vi "Initialize RT Main.vi"(8 "error in (no error)":errorcluster, 11 "OnCompile Settings":T1 {"XNET Settings"."Ghost"."FD ISO Mode" items=["ISO", "Non ISO", "ISO Legacy"]; "XNET Settings"."Ghost"."CAN I/O Mode" items=["CAN 2.0", "CAN FD", "CAN FD+BRS"]; "XNET Settings"."Ghost"."Termination" items=["Off", "On"]; "XNET Settings"."Primary"."FD ISO Mode" items=["ISO", "Non ISO", "ISO Legacy"]; "XNET Settings"."Primary"."CAN I/O Mode" items=["CAN 2.0", "CAN FD", "CAN FD+BRS"]; "XNET Settings"."Primary"."Termination" items=["Off", "On"]}) -> (0 "error out":errorcluster, 2 "FPGA Session":u32, 3 "Settings":T8[](array[typedef]) {"Port Info"."FD ISO Mode" items=["ISO", "Non ISO", "ISO Legacy"]; "Port Info"."CAN I/O Mode" items=["CAN 2.0", "CAN FD", "CAN FD+BRS"]; "Port Info"."Termination" items=["Off", "On"]})   [LabVIEW 2019, in "Ghost Bus Addon Engine.lvlib"]
uses:
  Ghost Bus Addon Engine.lvlib
  Types/RT Bus Settings.ctl
  Types/RT XNET Refs.ctl
  Addon Shared/Types/XNET Port Settings.ctl
  Types/RT Filter DVR Refs.ctl
  Addon Shared/Types/Exported.OnCompile.ctl
  Addon Shared/Types/XNET Settings.ctl
  Addon Shared/Types/Exported.Bus.Settings.ctl
  Addon Shared/Types/Exported.Frames.Settings.ctl
  Addon Shared/Types/Frame Settings.ctl
  Addon Shared/Types/986x.ctl
  Bitfile.Download.vi
  <vilib>/Utility/libraryn.llb/Check if File or Folder Exists.vi
  <vilib>/Utility/error.llb/Error Cluster From Error Code.vi
  <vilib>/rvi/Utilities/XML/nirviXML_GetValue.vi
  <vilib>/rvi/Utilities/XML/nirviXML_GetValue_String.vi
  <vilib>/xnet/xnet.llb/XNET Create Session.vi
  <vilib>/xnet/xnet.llb/XNET Create Session (Frame Output Stream).vi
  <vilib>/xnet/xnet.llb/XNET Create Session (Frame Input Stream).vi
  <vilib>/xnet/xnet.llb/XNET Create Session (Conversion).vi
  Addon Shared/Ghost Bus Addon Shared.lvlib
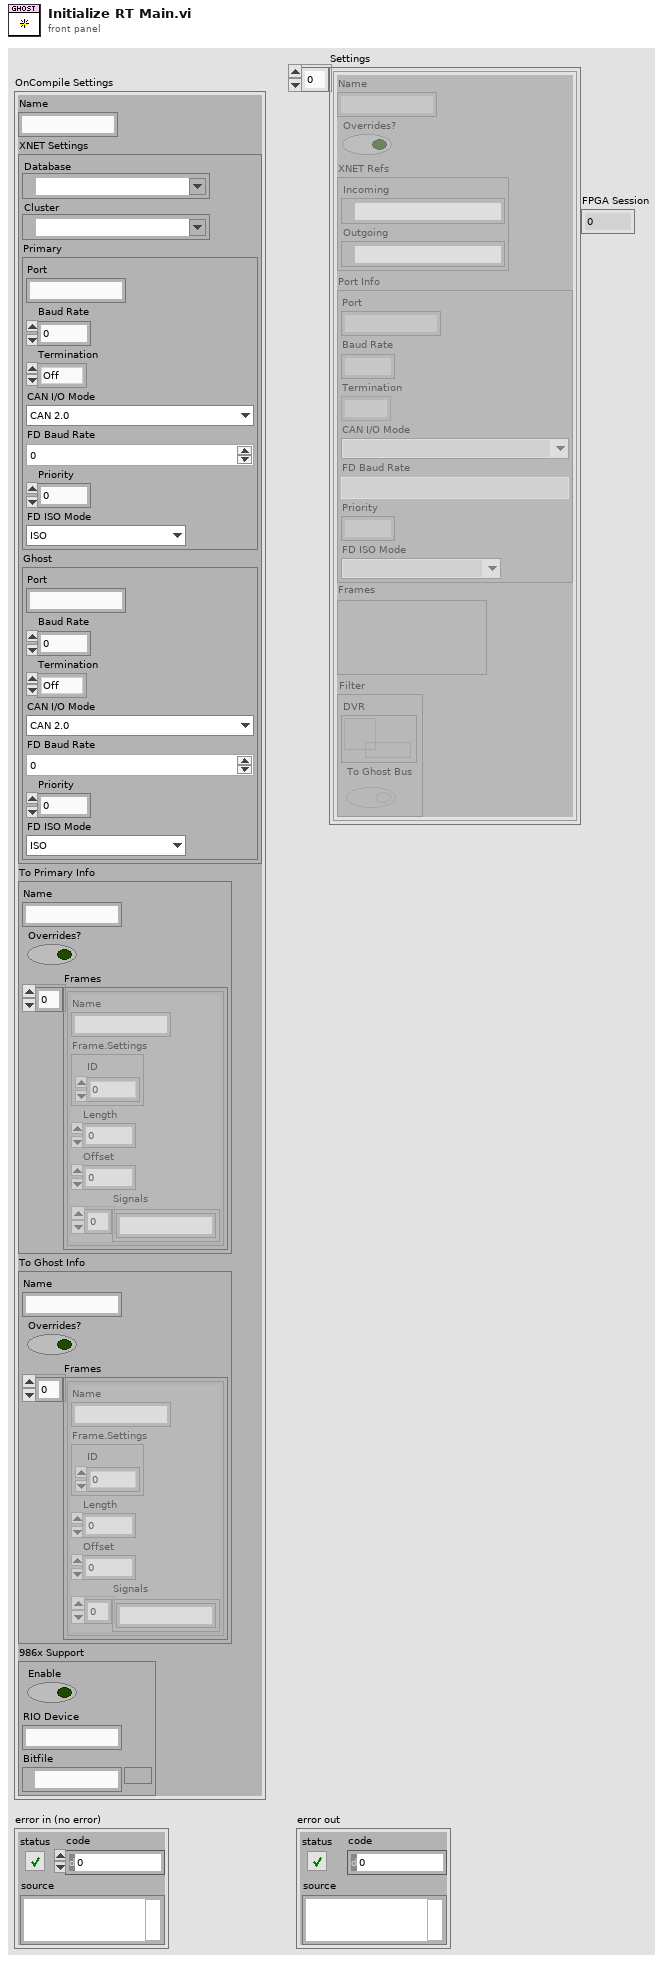
[diagram p1: front panel]
types:
  T1 = typedef "Ghost Bus Addon Shared.lvlib/Exported.OnCompile.ctl" = cluster{"Name":string, "XNET Settings":T2, "To Primary Info":T4, "To Ghost Info":T4, "986x Support":T7}
  T2 = typedef "Ghost Bus Addon Shared.lvlib/XNET Settings.ctl" = cluster{"Database":refnum<k21>, "Cluster":refnum<k21>, "Primary":T3, "Ghost":T3}
  T3 = typedef "Ghost Bus Addon Shared.lvlib/XNET Port Settings.ctl" = cluster{"Port":string, "Baud Rate":u64, "Termination":u32, "CAN I/O Mode":u32, "FD Baud Rate":u64, "Priority":i32, "FD ISO Mode":u32}
  T4 = typedef "Ghost Bus Addon Shared.lvlib/Exported.Bus.Settings.ctl" = cluster{"Name":string, "Overrides?":bool, "Frames":T5[]}
  T5 = typedef "Ghost Bus Addon Shared.lvlib/Exported.Frames.Settings.ctl" = cluster{"Name":string, "Frame.Settings":T6, "Length":i32, "Offset":i32, "Signals":string[]}
  T6 = typedef "Ghost Bus Addon Shared.lvlib/Frame Settings.ctl" = cluster{"ID":u32}
  T7 = typedef "Ghost Bus Addon Shared.lvlib/986x.ctl" = cluster{"Enable":bool, "RIO Device":string, "Bitfile":path}
  T8 = typedef "Ghost Bus Addon Engine.lvlib/RT Bus Settings.ctl" = cluster{"Name":string, "Overrides?":bool, "XNET Refs":T9, "Port Info":T3, "Frames":variant, "Filter":T10}
  T9 = typedef "Ghost Bus Addon Engine.lvlib/RT XNET Refs.ctl" = cluster{"Incoming":refnum<k21>, "Outgoing":refnum<k21>}
  T10 = typedef "Ghost Bus Addon Engine.lvlib/RT Filter DVR Refs.ctl" = cluster{"DVR":refnum<data-value>, "To Ghost Bus":bool}
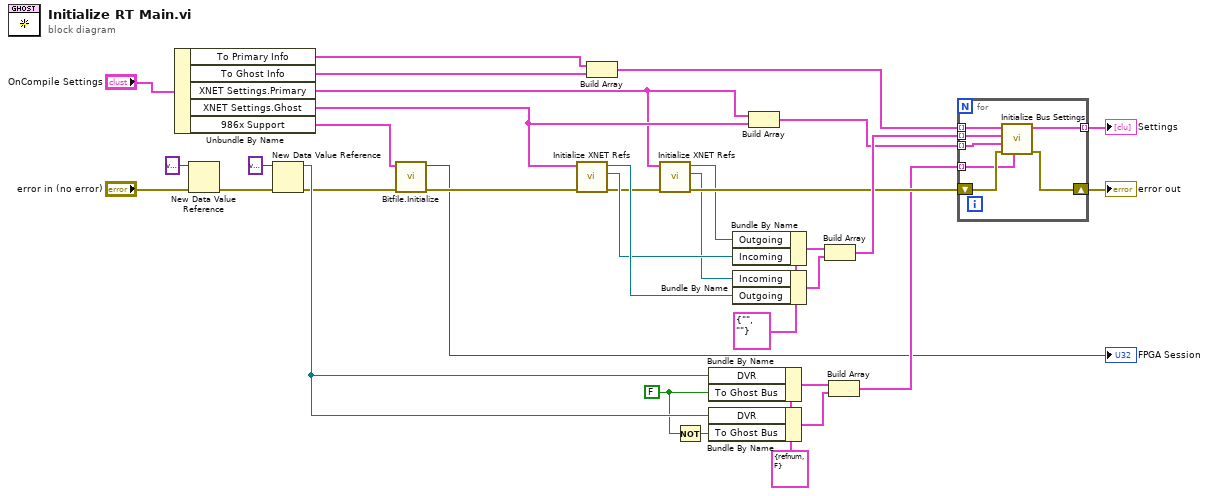
[diagram p0: block diagram]
diagram:
  w5 = FALSE ("To Ghost Bus")
  w9 = T10 {"DVR"=refnum, "To Ghost Bus"=FALSE} ("Filter DVRs")
  w29 = T9 {"Incoming"="", "Outgoing"=""} ("cluster")
  n1 = Unbundle By Name("OnCompile Settings") -> ("To Primary Info"=w22:T4, "To Ghost Info"=w23:T4, "XNET Settings.Primary"=w17:T3, "XNET Settings.Ghost"=w18:T3, "986x Support"=w2:T7)
  n2 = New Data Value Reference(data value=variant, error in="error in (no error)") -> (error out=w13:errorcluster)  [unwired: 1 out]
  n3 = New Data Value Reference(data value=variant, error in=w13) -> (data value reference=w11:refnum<data-value>, error out=w4:errorcluster)
  n4 = call "Bitfile.Initialize.vi"("error in (no error)"=w4, "FPGA Bitfile Settings"=w2) -> ("error out"=w3:errorcluster, "FPGA Session"=→"FPGA Session":u32)  [unwired: 8 in]
  n5 = call "Initialize XNET Refs.vi"("error in (no error)"=w3, "XNET Settings"=w18) -> ("error out"=w26:errorcluster, "Incoming"=w28:refnum<k21>, "Outgoing"=w30:refnum<k21>)  [unwired: 7 in]
  n6 = Build Array(w22, w23) -> (w24:T4[])
  n7 = call "Initialize XNET Refs.vi"("error in (no error)"=w26, "XNET Settings"=w17) -> ("error out"=w27:errorcluster, "Incoming"=w19:refnum<k21>, "Outgoing"=w20:refnum<k21>)  [unwired: 7 in]
  n8 = Not(x=w5) -> (.not. x?=w6:bool)
  n9 = Bundle By Name(cluster=w9, "DVR"=w11, "To Ghost Bus"=w5) -> (w10:T10)
  n10 = Bundle By Name(cluster=w9, "DVR"=w11, "To Ghost Bus"=w6) -> (w8:T10)
  n11 = Bundle By Name(cluster=w29, "Outgoing"=w20, "Incoming"=w28) -> (w31:T9)
  n12 = Bundle By Name(cluster=w29, "Incoming"=w19, "Outgoing"=w30) -> (w32:T9)
  n13 = Build Array(w17, w18) -> (w16:T3[])
  n14 = Build Array(w31, w32) -> (w33:T9[])
  n15 = Build Array(w10, w8) -> (w7:T10[])
  n16 = for {
    tunnel: w24 -> [w39] mode=indexing
    shift-right: [w40] -> w25
    shift-left: w27 -> [w41]
    tunnel: w33 -> [w38] mode=indexing
    tunnel: [w37] -> w34 mode=indexing
    tunnel: w16 -> [w36] mode=indexing
    tunnel: w7 -> [w35] mode=indexing
    n17 = call "Initialize Bus Settings.vi"("Filter DVRs"=w35, "error in (no error)"=w41, "XNET Settings"=w36, "XNET Refs"=w38, "Bus Info"=w39) -> ("error out"=w40:errorcluster, "Bus Settings"=w37:T8)  [unwired: 5 in]
  }
  "Settings" <- w34
  "error out" <- w25
